vi "Count Start.vi"(10 "Correction":i32, 11 "handle":i32) -> (2 "function return":i32, 3 "handle out":i32)   [LabVIEW 2022 SP3]
doc: "BOOL H11890API __stdcall H11890CountStart(HANDLE handle,BOOL Correction);"
uses:
  H11890api.dll
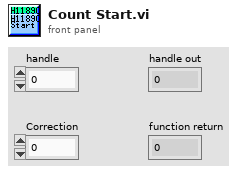
[diagram p1: front panel]
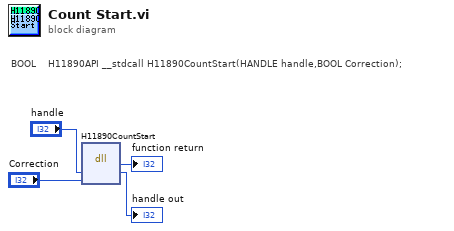
[diagram p0: block diagram]
diagram:
  # "BOOL \t\t\tH11890API __stdcall H11890CountStart(HANDLE handle,BOOL Correction);"
  n1 = dll-call lib="C:/Users/Public/OneDrive/Desktop/PMT_Project_folder/PMT_VIs/H11890api.dll" fn="H11890CountStart"("handle"="handle", "Correction"="Correction") -> ("Return"=→"function return":i32, "handle"=→"handle out":i32)  [unwired: 4 in, 2 out]
